vi "DataAveAnalysis.vi"(0 "CernoxI measured with a lock-in?":bool=TRUE, 1 "Title Name Array In":string[](array[string]), 2 "Cernox_I":dbl, 5 "2D Data Array In":dbl[][](array[numeric]), 7 "output cluster":T1={"Main Sweep"=0, "Steps Config:"={"total points:"=0, "Step Delay (s)"=0.0, "Ini Delay (s)"=0.0, "# of steps:"=0}, "Temperature Control (ITC 503):"={"GPIB ADR"=0, "Change Heater?"={"Heater?"=FALSE, "Heater"=0}, "Change Temp?"={"Change T?"=FALSE, "Set T (K)"=0.0}, "Cluster"={"Heat Auto?"=FALSE, "Manual Heat?"=FALSE, "Heater (%)"=0.0}, "Change PID?"={"Change PID?"=FALSE, "P"=0.0, "I"=0.0, "D"=0.0}, "Change Para?"=FALSE, "Sensor"=1}, "Temperature Control (LS 340):"={"GPIB ADR"=0, "From (K)"=0.0, "To (K)"=0.0, "Rate (K/min)"=0.0, "Delta T (0.08K)"=0.0, "Temp. Header"="", "T Display Control"={"Ch B"=FALSE, "Ch C"=FALSE, "Ch D"=FALSE}}, "Magnet Control (IPS 120-10)"={"Action"=0, "Standby (s)"=0.0, "Heater on (s)"=0.0, "Sweep Setup "=[], "GPIB ADR"=0, "Change Para?"=FALSE}, "Keithley 6221 :"=[], "Measuring Instruments : "=[], "Lock-In SR7265 :"=[], "Deascription of \nthis measurement"="", "Instruments Config:"=[], "LS372 Bridge : 2"=[{"GPIB"=0, "Excitation"=0, "Autorange?"=FALSE, "Range"=0, "Current"=0, "Voltage"=0, "DataHeader"="Rx;Ry"}], "Magnet Control (CS4) 2"={"Action"=1, "Standby (s)"=0.0, "Heater on (s)"=300.0, "Sweep Setup "=[], "GPIB ADR"=0, "Change Para?"=FALSE}} {"Magnet Control (CS4) 2"."GPIB ADR" items=["None"=0, "25"=25]; "Magnet Control (CS4) 2"."Sweep Setup"."Rate in Range (T/min)" min=0.001 max=0.5 step=0.001; "Magnet Control (CS4) 2"."Sweep Setup"."Hold(min)" min=0.0; "Magnet Control (CS4) 2"."Sweep Setup"."Set Point (T)" min=-9.0 max=9.0 step=0.001; "Magnet Control (CS4) 2"."Action" items=["Up", "Down", "Pause", "Zero"]; "LS372 Bridge : 2"."Voltage" items=["2.00 uV"=1, "6.32 uV"=2, "20.0 uV"=3, "63.2 uV"=4, "200 uV"=5, "632 uV"=6, "2.0 mV"=7, "6.32 mV"=8]; "LS372 Bridge : 2"."Current" items=["1.00 pA"=1, "3.16 pA"=2, "10.0 pA"=3, "31.6 pA"=4, "100 pA"=5, "316 pA"=6, "1.00 nA"=7, "3.16 nA"=8, "10 nA"=9, "31.6 nA"=10, "100 nA"=11, "316 nA"=12, "1.00 uA"=13, "3.16 uA"=14, "10.0 uA"=15, "31.6 uA"=16, "100 uA"=17, "316 uA"=18, "1.00 mA"=19, "3.16 mA"=20, "10.0 mA"=21, "31.6 mA"=22]; "LS372 Bridge : 2"."Range" items=["2.0 m"=1, "6.32 m"=2, "20.0 m"=3, "63.2 m"=4, "200 m"=5, "632 m"=6, "2.00"=7, "6.32"=8, "20.0"=9, "63.2"=10, "200"=11, "632"=12, "2.00 k"=13, "6.32 k"=14, "20.0 k"=15, "63.2 k"=16, "200 k"=17, "632 k"=18, "2.00 M"=19, "6.32 M"=20, "20.0 M"=21, "63.2 M"=22]; "LS372 Bridge : 2"."Excitation" items=["Voltage", "Current"]; "LS372 Bridge : 2"."GPIB" items=["None"=0, "9"=9]; "Main Sweep" items=["Time", "DC Current", "Delta Current", "Pulse Delta Current", "Sine Current", "Lock-in Vosc"]; "Temperature Control (ITC 503):"."Sensor" items=["T2", "T3"]; "Magnet Control (IPS 120-10)"."Action" items=["Hold", "To Set point", "To Zero", "Clamp"]; "Keithley 6221 :"."Sweep Mode" items=["Linear", "Log", "Exp", "Inverse", "Manual"]}, 9 "# of Discarded pts":i32, 11 "error in":errorcluster, 12 "Cernox T Fitting Control":T2) -> (3 "Title Name Array Out":string[](array[string]), 4 "output cluster 2":T1={"Main Sweep"=0, "Steps Config:"={"total points:"=0, "Step Delay (s)"=0.0, "Ini Delay (s)"=0.0, "# of steps:"=0}, "Temperature Control (ITC 503):"={"GPIB ADR"=0, "Change Heater?"={"Heater?"=FALSE, "Heater"=0}, "Change Temp?"={"Change T?"=FALSE, "Set T (K)"=0.0}, "Cluster"={"Heat Auto?"=FALSE, "Manual Heat?"=FALSE, "Heater (%)"=0.0}, "Change PID?"={"Change PID?"=FALSE, "P"=0.0, "I"=0.0, "D"=0.0}, "Change Para?"=FALSE, "Sensor"=1}, "Temperature Control (LS 340):"={"GPIB ADR"=0, "From (K)"=0.0, "To (K)"=0.0, "Rate (K/min)"=0.0, "Delta T (0.08K)"=0.0, "Temp. Header"="", "T Display Control"={"Ch B"=FALSE, "Ch C"=FALSE, "Ch D"=FALSE}}, "Magnet Control (IPS 120-10)"={"Action"=0, "Standby (s)"=0.0, "Heater on (s)"=0.0, "Sweep Setup "=[], "GPIB ADR"=0, "Change Para?"=FALSE}, "Keithley 6221 :"=[], "Measuring Instruments : "=[], "Lock-In SR7265 :"=[], "Deascription of \nthis measurement"="", "Instruments Config:"=[], "LS372 Bridge : 2"=[{"GPIB"=0, "Excitation"=0, "Autorange?"=FALSE, "Range"=0, "Current"=0, "Voltage"=0, "DataHeader"="Rx;Ry"}], "Magnet Control (CS4) 2"={"Action"=1, "Standby (s)"=0.0, "Heater on (s)"=300.0, "Sweep Setup "=[], "GPIB ADR"=0, "Change Para?"=FALSE}} {"Magnet Control (CS4) 2"."GPIB ADR" items=["None"=0, "25"=25]; "Magnet Control (CS4) 2"."Sweep Setup"."Rate in Range (T/min)" min=0.001 max=0.5 step=0.001; "Magnet Control (CS4) 2"."Sweep Setup"."Hold(min)" min=0.0; "Magnet Control (CS4) 2"."Sweep Setup"."Set Point (T)" min=-9.0 max=9.0 step=0.001; "Magnet Control (CS4) 2"."Action" items=["Up", "Down", "Pause", "Zero"]; "LS372 Bridge : 2"."Voltage" items=["2.00 uV"=1, "6.32 uV"=2, "20.0 uV"=3, "63.2 uV"=4, "200 uV"=5, "632 uV"=6, "2.0 mV"=7, "6.32 mV"=8]; "LS372 Bridge : 2"."Current" items=["1.00 pA"=1, "3.16 pA"=2, "10.0 pA"=3, "31.6 pA"=4, "100 pA"=5, "316 pA"=6, "1.00 nA"=7, "3.16 nA"=8, "10 nA"=9, "31.6 nA"=10, "100 nA"=11, "316 nA"=12, "1.00 uA"=13, "3.16 uA"=14, "10.0 uA"=15, "31.6 uA"=16, "100 uA"=17, "316 uA"=18, "1.00 mA"=19, "3.16 mA"=20, "10.0 mA"=21, "31.6 mA"=22]; "LS372 Bridge : 2"."Range" items=["2.0 m"=1, "6.32 m"=2, "20.0 m"=3, "63.2 m"=4, "200 m"=5, "632 m"=6, "2.00"=7, "6.32"=8, "20.0"=9, "63.2"=10, "200"=11, "632"=12, "2.00 k"=13, "6.32 k"=14, "20.0 k"=15, "63.2 k"=16, "200 k"=17, "632 k"=18, "2.00 M"=19, "6.32 M"=20, "20.0 M"=21, "63.2 M"=22]; "LS372 Bridge : 2"."Excitation" items=["Voltage", "Current"]; "LS372 Bridge : 2"."GPIB" items=["None"=0, "9"=9]; "Main Sweep" items=["Time", "DC Current", "Delta Current", "Pulse Delta Current", "Sine Current", "Lock-in Vosc"]; "Temperature Control (ITC 503):"."Sensor" items=["T2", "T3"]; "Magnet Control (IPS 120-10)"."Action" items=["Hold", "To Set point", "To Zero", "Clamp"]; "Keithley 6221 :"."Sweep Mode" items=["Linear", "Log", "Exp", "Inverse", "Manual"]}, 6 "2D Data ArrayOut":dbl[][](array[numeric]), 10 "2D Data  Analysis":dbl[][](array[numeric]), 14 "Title Name Before Std":string[](array[string]), 15 "error out":errorcluster)   [LabVIEW 2012]
uses:
  <vilib>/Analysis/NI_AALBase.lvlib
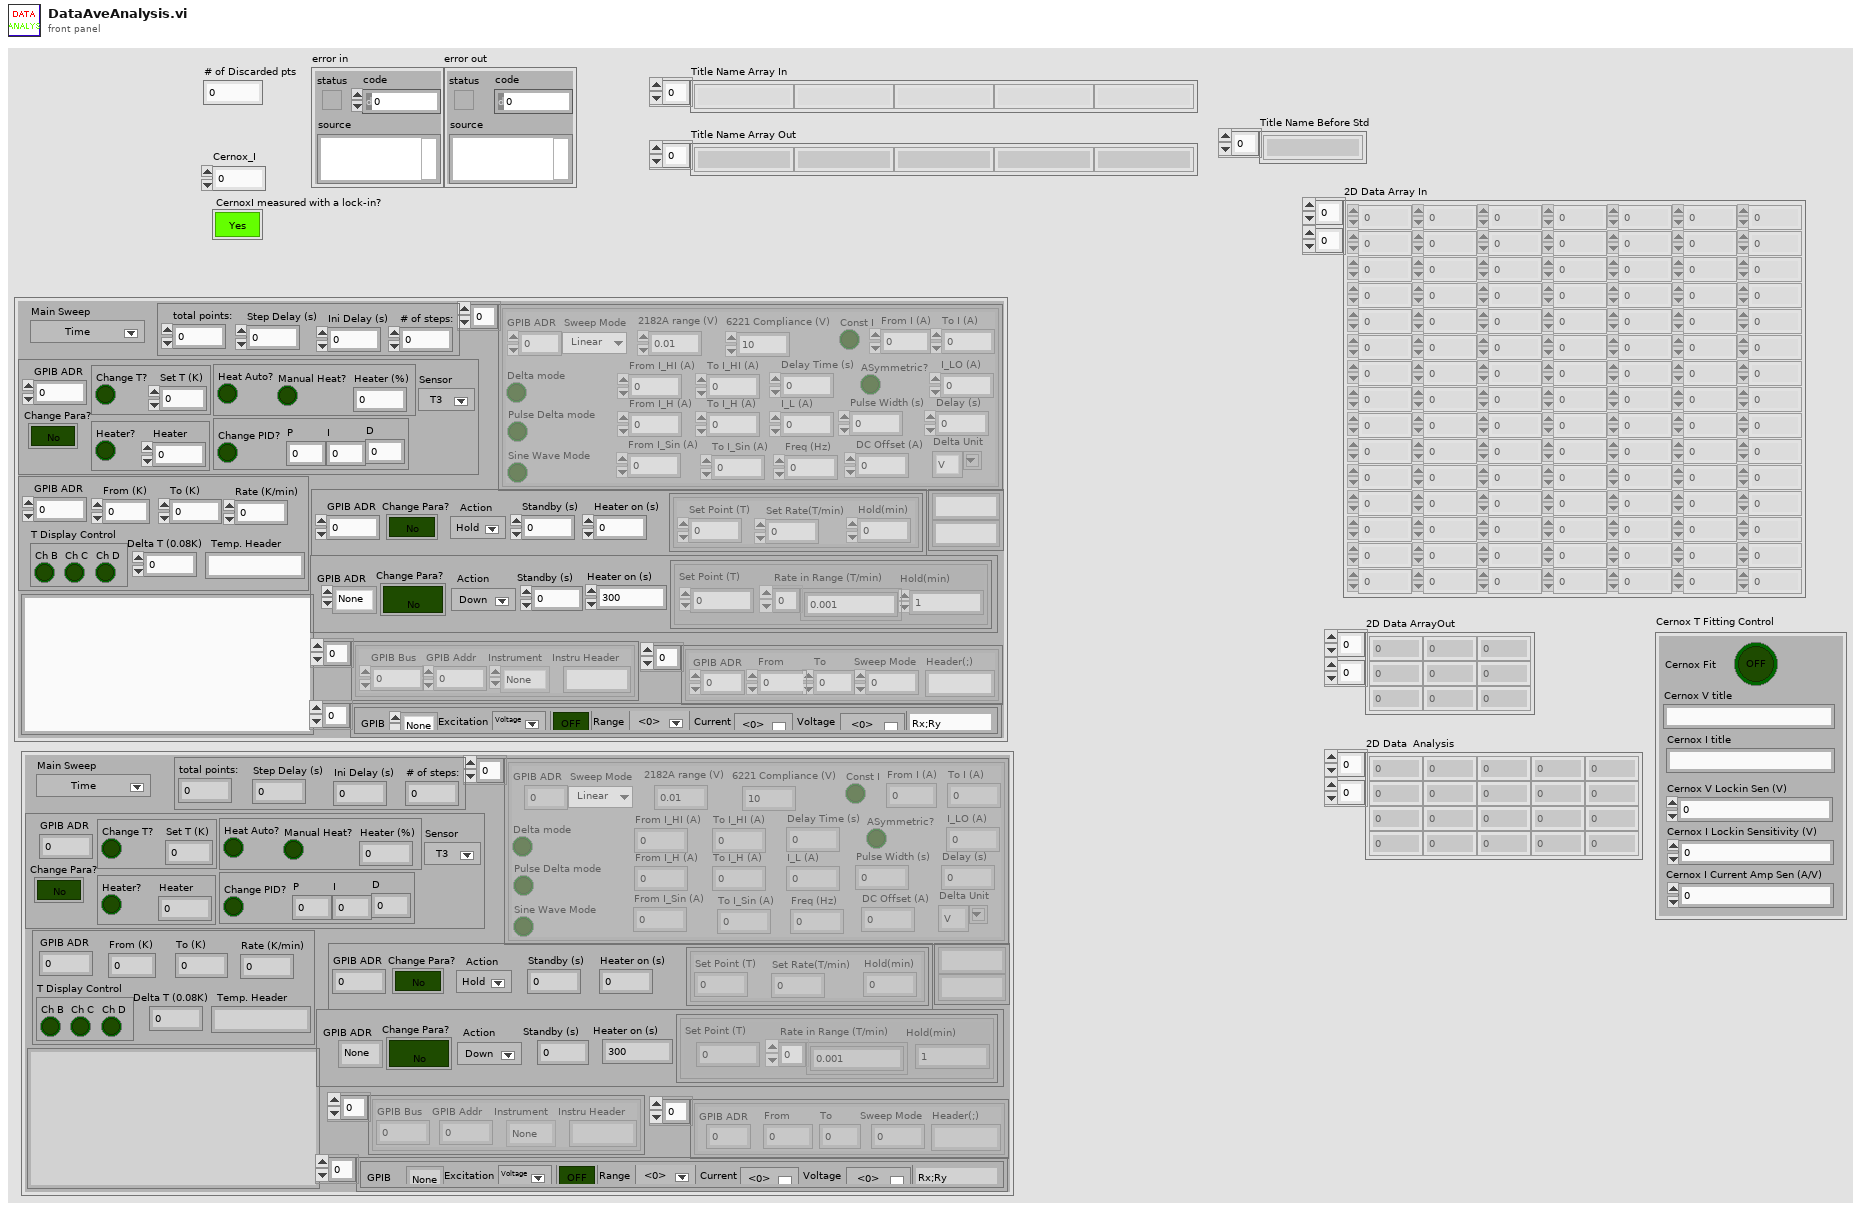
[diagram p1: front panel]
types:
  T1 = cluster{"Main Sweep":u8, "Steps Config:":cluster{"total points:":u32, "Step Delay (s)":dbl, "Ini Delay (s)":dbl, "# of steps:":u32}, "Temperature Control (ITC 503):":cluster{"GPIB ADR":u16, "Change Heater?":cluster{"Heater?":bool, "Heater":u8}, "Change Temp?":cluster{"Change T?":bool, "Set T (K)":dbl}, "Cluster":cluster{"Heat Auto?":bool, "Manual Heat?":bool, "Heater (%)":dbl}, "Change PID?":cluster{"Change PID?":bool, "P":dbl, "I":dbl, "D":dbl}, "Change Para?":bool, "Sensor":u16}, "Temperature Control (LS 340):":cluster{"GPIB ADR":u16, "From (K)":dbl, "To (K)":dbl, "Rate (K/min)":dbl, "Delta T (0.08K)":dbl, "Temp. Header":string, "T Display Control":cluster{"Ch B":bool, "Ch C":bool, "Ch D":bool}}, "Magnet Control (IPS 120-10)":cluster{"Action":u16, "Standby (s)":dbl, "Heater on (s)":dbl, "Sweep Setup ":cluster{"Set Point (T)":dbl, "Set Rate(T/min)":dbl, "Hold(min)":dbl}[], "GPIB ADR":u16, "Change Para?":bool}, "Keithley 6221 :":cluster{"Delta mode":bool, "Const I":bool, "Pulse Delta mode":bool, "Sine Wave Mode":bool, "From I_HI (A)":dbl, "From I (A)":dbl, "I_LO (A)":dbl, "From I_H (A)":dbl, "I_L (A)":dbl, "Freq (Hz)":dbl, "From I_Sin (A)":dbl, "DC Offset (A)":dbl, "Delay Time (s)":dbl, "Pulse Width (s)":dbl, "Delay (s)":dbl, "To I (A)":dbl, "ASymmetric?":bool, "To I_HI (A)":dbl, "To I_H (A)":dbl, "To I_Sin (A)":dbl, "GPIB ADR":u16, "Sweep Mode":u8, "Delta Unit":string, "2182A range (V)":dbl, "6221 Compliance (V)":dbl}[], "Measuring Instruments : ":cluster{"GPIB Bus":dbl, "GPIB Addr":dbl, "Instrument":enum16{"None", "HP34401DMM", "Lockin 7265", "HP3456/7A", "HP3478A", "HP3325FG", "Keithley2182A"}, "Instru Header":string}[], "Lock-In SR7265 :":cluster{"GPIB ADR":u16, "From":dbl, "To":dbl, "Header(;)":string, "Sweep Mode":u8}[], "Deascription of \nthis measurement":string, "Instruments Config:":string[][], "LS372 Bridge : 2":cluster{"GPIB":u16, "Excitation":u16, "Autorange?":bool, "Range":u16, "Current":u16, "Voltage":u16, "DataHeader":string}[], "Magnet Control (CS4) 2":cluster{"Action":u16, "Standby (s)":dbl, "Heater on (s)":dbl, "Sweep Setup ":cluster{"Set Point (T)":dbl, "Hold(min)":dbl, "Rate in Range (T/min)":dbl[]}[], "GPIB ADR":u16, "Change Para?":bool}}
  T2 = cluster{"Cernox V title":string, "Cernox I title":string, "Cernox V Lockin Sen (V)":dbl, "Cernox I Lockin Sensitivity (V)":dbl, "Cernox I Current Amp Sen (A/V)":dbl, "Cernox Fit":bool}
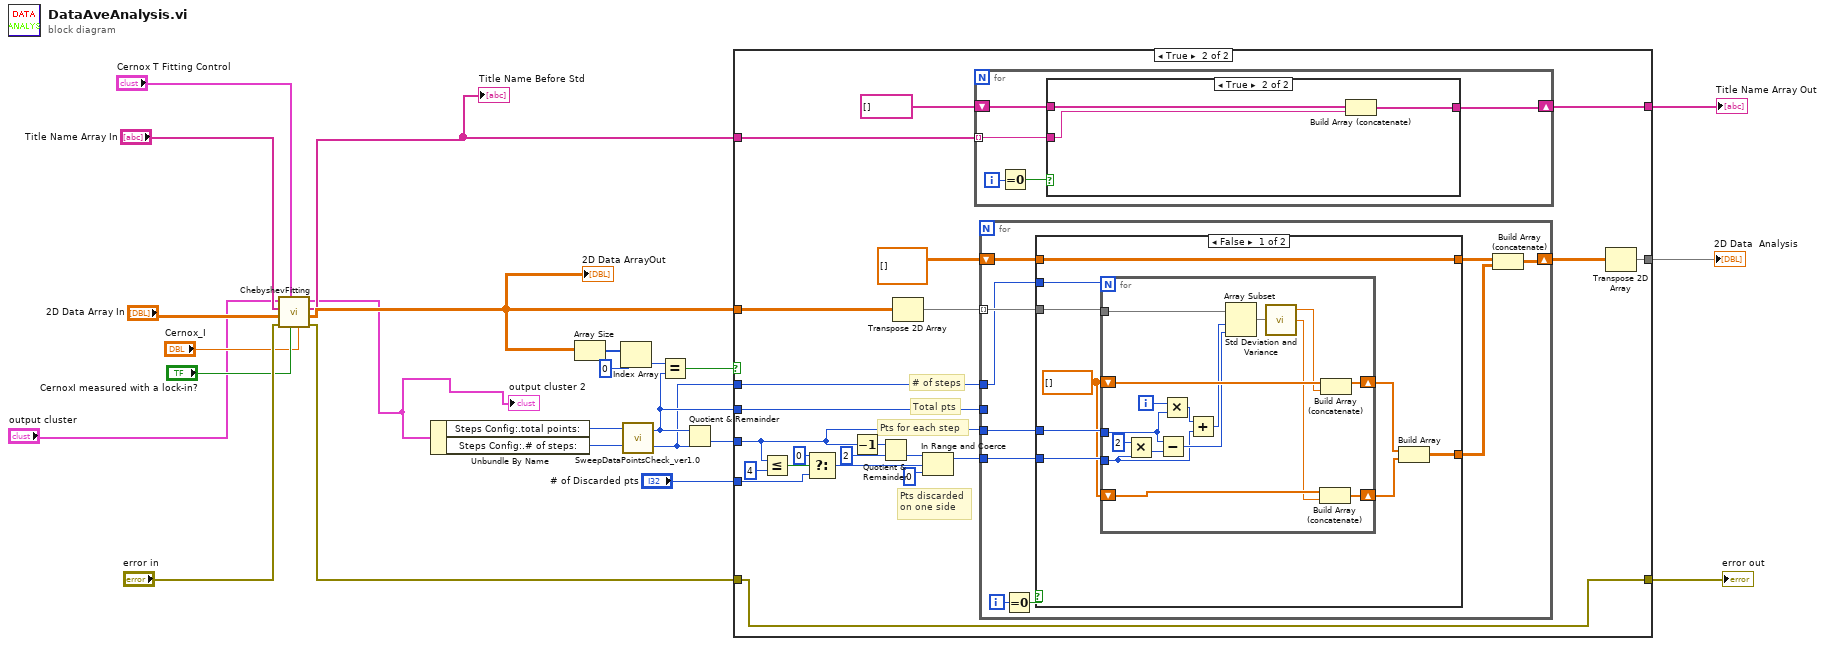
[diagram p0: block diagram]
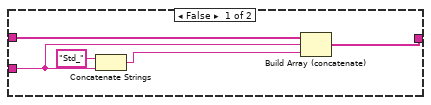
[diagram p3: hidden frame]
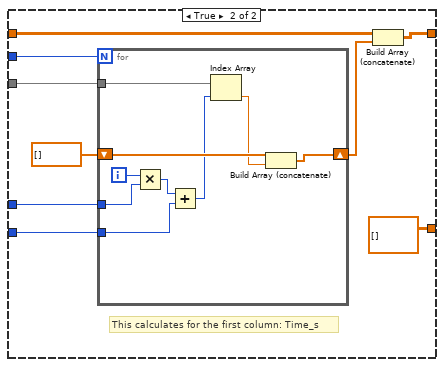
[diagram p4: hidden frame]
diagram:
  n1 = call "ChebyshevFitting.vi"("Cernox_I"="Cernox_I", "CernoxI measured with a lock-in?"="CernoxI measured with a lock-in?", "Cernox T Fitting Control"="Cernox T Fitting Control", "error in"="error in", "2D Data Array In"="2D Data Array In", "Title Name Array In"="Title Name Array In", "output cluster"="output cluster") -> ("error out"=w6:errorcluster, "2D Data ArrayOut"=w8:dbl[][], "Title Name Array Out"=w7:string[], "output cluster 2"=w1:T1)  [unwired: 1 in]
  "2D Data ArrayOut" <- w8
  "Title Name Before Std" <- w7
  "output cluster 2" <- w1
  n2 = Unbundle By Name(w1) -> ("Steps Config:.total points:"=w24:u32, "Steps Config:.# of steps:"=w23:u32)
  n3 = Array Size(array=w8) -> (size(s)=w22:i32[])
  n4 = Index Array(array=w22, index=0) -> (element=w20:i32)
  n5 = call "SweepDataPointsCheck_ver1.0.vi"("Input # of sweep steps:"=w23, "Input # of total points:"=w24) -> ("Output # of sweep steps:"=w14:u32, "Output # of total points:"=w16:u32)
  n6 = Equal?(x=w20, y=w16) -> (x = y?=w19:bool)
  n7 = Quotient & Remainder(x=w16, y=w14) -> (floor(x/y)=w18:u32)  [unwired: 1 out]
  n8 = case shown="True" w19 {
    tunnel: w18 -> [_ w38]
    tunnel: "# of Discarded pts" -> [_ w42]
    tunnel: w6 -> [w27 w32]
    tunnel: [w27 w32] -> w17
    tunnel: w8 -> [w25 w48]
    tunnel: w16 -> [_ w45]
    tunnel: w14 -> [_ w35]
    tunnel: [w25 w33] -> w13
    tunnel: w7 -> [w26 w30]
    tunnel: [w26 w28] -> w12
    frame False {
    }
    frame True {
      # "# of steps"
      # "Pts for each step"
      # "Total pts"
      # "Pts discarded\non one side"
      n9 = Less Or Equal?(x=w38, y=u32 4) -> (x <= y?=w43:bool)
      n10 = Select(t=0, s=w43, f=w42) -> (s? t:f=w41:i32)
      n11 = Decrement(x=w38) -> (x-1=w36:u32)
      n12 = Quotient & Remainder(x=w36, y=u32 2) -> (floor(x/y)=w39:u32)  [unwired: 1 out]
      n13 = Transpose 2D Array(2D array=w48) -> (transposed array=w47:dbl[][])
      n14 = In Range and Coerce(upper limit=w39, x=w41, lower limit=u32 0) -> (coerced(x)=w46:u32)  [unwired: 1 out]
      n15 = for {
        tunnel: w30 -> [w52] mode=indexing
        shift-right: [w50] -> w28
        shift-left: string[] [] ("Title Name Array In") -> [w51]
        i -> [w54]
        n16 = Equal To 0?(x=w54) -> (x = 0?=w53:bool)
        n17 = case shown="True" w53 {
          tunnel: w52 -> [w56 w61]
          tunnel: w51 -> [w58 w62]
          tunnel: [w57 w60] -> w50
          frame False {
            n18 = Concatenate Strings("Std_" ("string"), w56) -> (w55:string)
            n19 = Build Array (concatenate)(w58, w56, w55) -> (w57:string[])
          }
          frame True {
            n20 = Build Array (concatenate)(w62, w61) -> (w60:string[])
          }
        }
      }
      n21 = for {
        tunnel: w47 -> [w72] mode=indexing
        tunnel: w46 -> [w67]
        tunnel: w45 -> [_]
        tunnel: w38 -> [w68]
        tunnel: w35 -> [w69]
        shift-right: [w64] -> w31
        shift-left: dbl[][] [] -> [w66]
        i -> [w71]
        n22 = Equal To 0?(x=w71) -> (x = 0?=w70:bool)
        n23 = case shown="False" w70 {
          tunnel: w72 -> [w79 w106]
          tunnel: w69 -> [w80 w105]
          tunnel: w68 -> [w78 w103]
          tunnel: w67 -> [w77 w102]
          tunnel: w66 -> [w81 w100]
          tunnel: [w81 w98] -> w65
          tunnel: [w73 dbl[][] []] -> w63
          frame False {
            w76 = dbl[] []
            n24 = for {
              N: w80 -> [_]
              tunnel: w79 -> [w97]
              shift-right: [w95] -> w75
              shift-left: w76 -> [w96]
              tunnel: w78 -> [w91]
              tunnel: w77 -> [w84]
              shift-right: [w85] -> w74
              shift-left: w76 -> [w87]
              i -> [w94]
              n25 = Multiply(x=u32 2, y=w84) -> (x*y=w82:u32)
              n26 = Subtract(x=w91, y=w82) -> (x-y=w90:u32)
              n27 = Multiply(x=w94, y=w91) -> (x*y=w93:u32)
              n28 = Add(x=w93, y=w84) -> (x+y=w92:u32)
              n29 = Array Subset(array=w97, index=w92, length=w90) -> (w89:dbl[])
              n30 = call <vilib>:"Std Deviation and Variance.vi"("X"=w89) -> ("mean"=w88:dbl, "standard deviation"=w86:dbl)  [unwired: 1 in, 1 out]
              n31 = Build Array (concatenate)(w87, w86) -> (w85:dbl[])
              n32 = Build Array (concatenate)(w96, w88) -> (w95:dbl[])
            }
            n33 = Build Array(w75, w74) -> (w73:dbl[][])
          }
          frame True {
            # "This calculates for the first column: Time_s"
            n34 = for {
              N: w105 -> [_]
              tunnel: w106 -> [w115]
              shift-right: [w113] -> w99
              shift-left: dbl[] [] -> [w114]
              tunnel: w103 -> [w111]
              tunnel: w102 -> [w109]
              i -> [w112]
              n35 = Multiply(x=w112, y=w111) -> (x*y=w110:u32)
              n36 = Add(x=w110, y=w109) -> (x+y=w108:u32)
              n37 = Index Array(array=w115, index=w108) -> (element=w107:dbl)
              n38 = Build Array (concatenate)(w114, w107) -> (w113:dbl[])
            }
            n39 = Build Array (concatenate)(w100, w99) -> (w98:dbl[][])
          }
        }
        n40 = Build Array (concatenate)(w65, w63) -> (w64:dbl[][])
      }
      n41 = Transpose 2D Array(2D array=w31) -> (transposed array=w33:dbl[][])
    }
  }
  "error out" <- w17
  "2D Data  Analysis" <- w13
  "Title Name Array Out" <- w12
